vi "Poly Fit (Second Degree).vi"(0 "Reference":dbl[](array[numeric]), 11 "Actual":dbl[](array[numeric])) -> (8 "A0x2,A1x,A3":dbl[](array[numeric]))   [LabVIEW 2013]
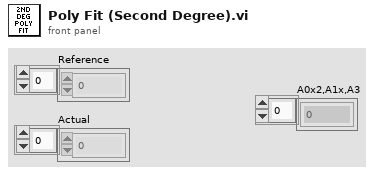
[diagram p1: front panel]
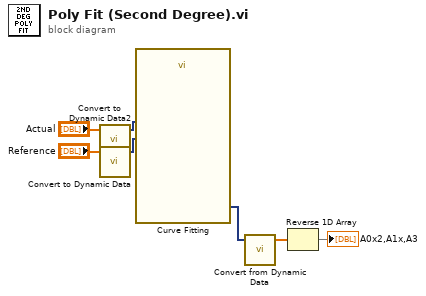
[diagram p0: block diagram]
diagram:
  n1 = call "Convert to Dynamic Data2"("Array"="Actual") -> ("Dynamic Data Type"=w6:dynamicdata)  [unwired: 3 in]
  n2 = call "Convert to Dynamic Data"("Array"="Reference") -> ("Dynamic Data Type"=w7:dynamicdata)  [unwired: 3 in]
  n3 = call "Curve Fitting"("Locations"=w7, "Signals"=w6) -> ("polynomial coefficients"=w5:dynamicdata)  [unwired: 5 in, 4 out]
  n4 = call "Convert from Dynamic Data"("Dynamic Data Type"=w5) -> ("Array"=w2:dbl[])  [unwired: 3 in]
  n5 = Reverse 1D Array(array=w2) -> (reversed array=→"A0x2,A1x,A3":dbl[])
